vi "SetTriggerSource.vi"(8 "error in (no error)":errorcluster, 10 "Settings.Trigger":T1, 11 "Point Grey Camera in":refnum<class "Point Grey Camera.lvclass">) -> (0 "error out":errorcluster, 2 "Settings.Trigger  out":T1, 3 "Point Grey Camera out":refnum<class "Point Grey Camera.lvclass">)   [LabVIEW 2020, in "Point Grey Camera.lvclass"]
uses:
  Point Grey Camera.lvclass
  OnOffTypeDef.ctl
  Point Grey Camera.lvclass/Point Grey Camera.ctl
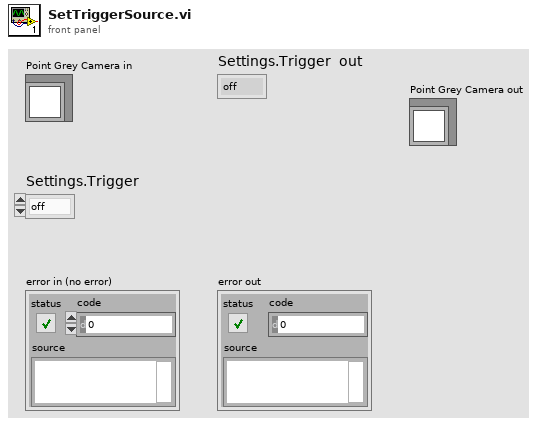
[diagram p1: front panel]
types:
  T1 = typedef "OnOffTypeDef.ctl" = enum16{"off", "on"}
  T2 = typedef "TriggerSource_TypDEF.ctl" = cluster{"Software":string, "External":string, "Execute":string}
  T3 = typedef "IMAQdx.ctl" = refnum<k21>
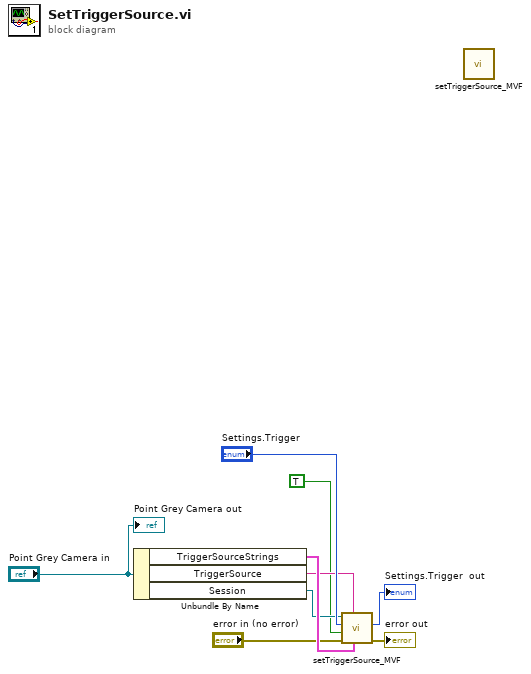
[diagram p0: block diagram]
diagram:
  n1 = Unbundle By Name("Point Grey Camera in") -> ("TriggerSourceStrings"=w8:T2, "TriggerSource"=w5:string, "Session"=w6:T3)
  n2 = call "setTriggerSource_MVF.vi"("TriggerSourceStrings"=w8, "TrigerModeName"=w5, "error in"="error in (no error)", "cam connected"=TRUE, "Settings.Trigger"="Settings.Trigger", "Session"=w6) -> ("error out"=→"error out":errorcluster, "Settings.Trigger  out"=→"Settings.Trigger  out":T1)  [unwired: 4 in]
  n3 = call "setTriggerSource_MVF.vi"() -> ()  [unwired: 10 in, 2 out]
  "Point Grey Camera out" <- "Point Grey Camera in"
